vi "TwoBallShortAuton.vi"(11 "Intake Suck at Beginning?":bool) -> ()   [LabVIEW 2013]
uses:
  <vilib>/Rock Robotics/WPI/SafetyOutput/WPI_SafetyOutputConfigMenu.ctl
  <vilib>/Rock Robotics/WPI/Solenoid/WPI_SolenoidValue.ctl
  <vilib>/Rock Robotics/WPI/RobotDrive/WPI_RobotDriveGetSetRefNum.vi
  <vilib>/Rock Robotics/WPI/Solenoid/WPI_SolenoidSetEnum.vi
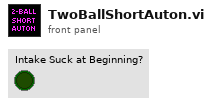
[diagram p1: front panel]
types:
  T1 = typedef "WPI_SafetyOutputConfigMenu.ctl" = enum16{"Enable", "Disable"}
  T2 = typedef "WPI_RobotDriveDevRef.ctl" = cluster{"DevStatus":errorcluster, "Motors[]":T3[], "Square Inputs":bool, "Max Output":dbl, "Isochronous":bool}
  T3 = typedef "WPI_MotorControlDeviceRef.ctl" = cluster{"DeviceStatus":errorcluster, "Type":enum16{"PWM", "CAN"}, "PWM":cluster{"Digital Module":T4, "PWM Channel":T5, "DeadBand":T6}, "CAN":cluster{"Device Number":u8, "Control Mode":T7, "Semaphore":T8, "Max Vout":dbl}, "Invert":bool, "TransformRef":T9, "InvTransformRef":T9}
  T4 = typedef "FPGA_TypedefDigitalModule.ctl" = enum16{"Digital Module 1", "Digital Module 2"}
  T5 = typedef "FPGA_DIOPWMChannel.ctl" = enum8{"PWM 1", "PWM 2", "PWM 3", "PWM 4", "PWM 5", "PWM 6", "PWM 7", "PWM 8", "PWM 9", "PWM 10", "Invalid"}
  T6 = typedef "WPI_PWMDeadband.ctl" = cluster{"Name":string, "maxPositivePwm":i32, "minPositivePwm":i32, "centerPwm":i32, "maxNegativePwm":i32, "minNegativePwm":i32, "angularRange":u16}
  T7 = typedef "WPI_CANJaguar_ControlMode.ctl" = enum8{"Percent VBus", "Current", "Speed", "Position", "Voltage"}
  T8 = typedef "Semaphore RefNum" = refnum<k1>
  T9 = typedef "WPI_PWMTransform_ConPane.ctl" = refnum<vi>
  T10 = typedef "WPI_DigitalInputDevRef.ctl" = cluster{"DevStatus":errorcluster, "DIO Channel":T11, "Digital Module":T4}
  T11 = typedef "FPGA_DIOChannel.ctl" = enum8{"DIO 1", "DIO 2", "DIO 3", "DIO 4", "DIO 5", "DIO 6", "DIO 7", "DIO 8", "DIO 9", "DIO 10", "DIO 11", "DIO 12", "DIO 13", "DIO 14", "Invalid"}
  T12 = typedef "WPI_SolenoidDevRef.ctl" = cluster{"DevStatus":errorcluster, "Solenoid Module":T13, "Forward Solenoid Channel":T14, "Reverse Solenoid Channel":T14}
  T13 = typedef "FPGA_TypedefSolenoidModule.ctl" = enum16{"Solenoid Module 1", "Solenoid Module 2"}
  T14 = typedef "WPI_SolenoidChannel.ctl" = enum8{"Solenoid 1", "Solenoid 2", "Solenoid 3", "Solenoid 4", "Solenoid 5", "Solenoid 6", "Solenoid 7", "Solenoid 8", "Invalid"}
  T15 = typedef "WPI_EncoderDevRef.ctl" = cluster{"DevStatus":errorcluster, "EncoderIndex":T16, "CounterIndex":T17, "DistancePerCount":dbl, "Decoding Type":T18}
  T16 = typedef "FPGA_EncoderIdx.ctl" = enum8{"Enc 0", "Enc 1", "Enc 2", "Enc 3", "Invalid"}
  T17 = typedef "FPGA_CounterCtrSystemIndex.ctl" = enum8{"Ctr 0", "Ctr 1", "Ctr 2", "Ctr 3", "Ctr 4", "Ctr 5", "Ctr 6", "Ctr 7", "Invalid"}
  T18 = typedef "WPI_EncoderType.ctl" = enum16{"1x", "2x", "4x"}
  T19 = typedef "WPI_SolenoidValue.ctl" = enum16{"Off", "On", "Forward", "Reverse"}
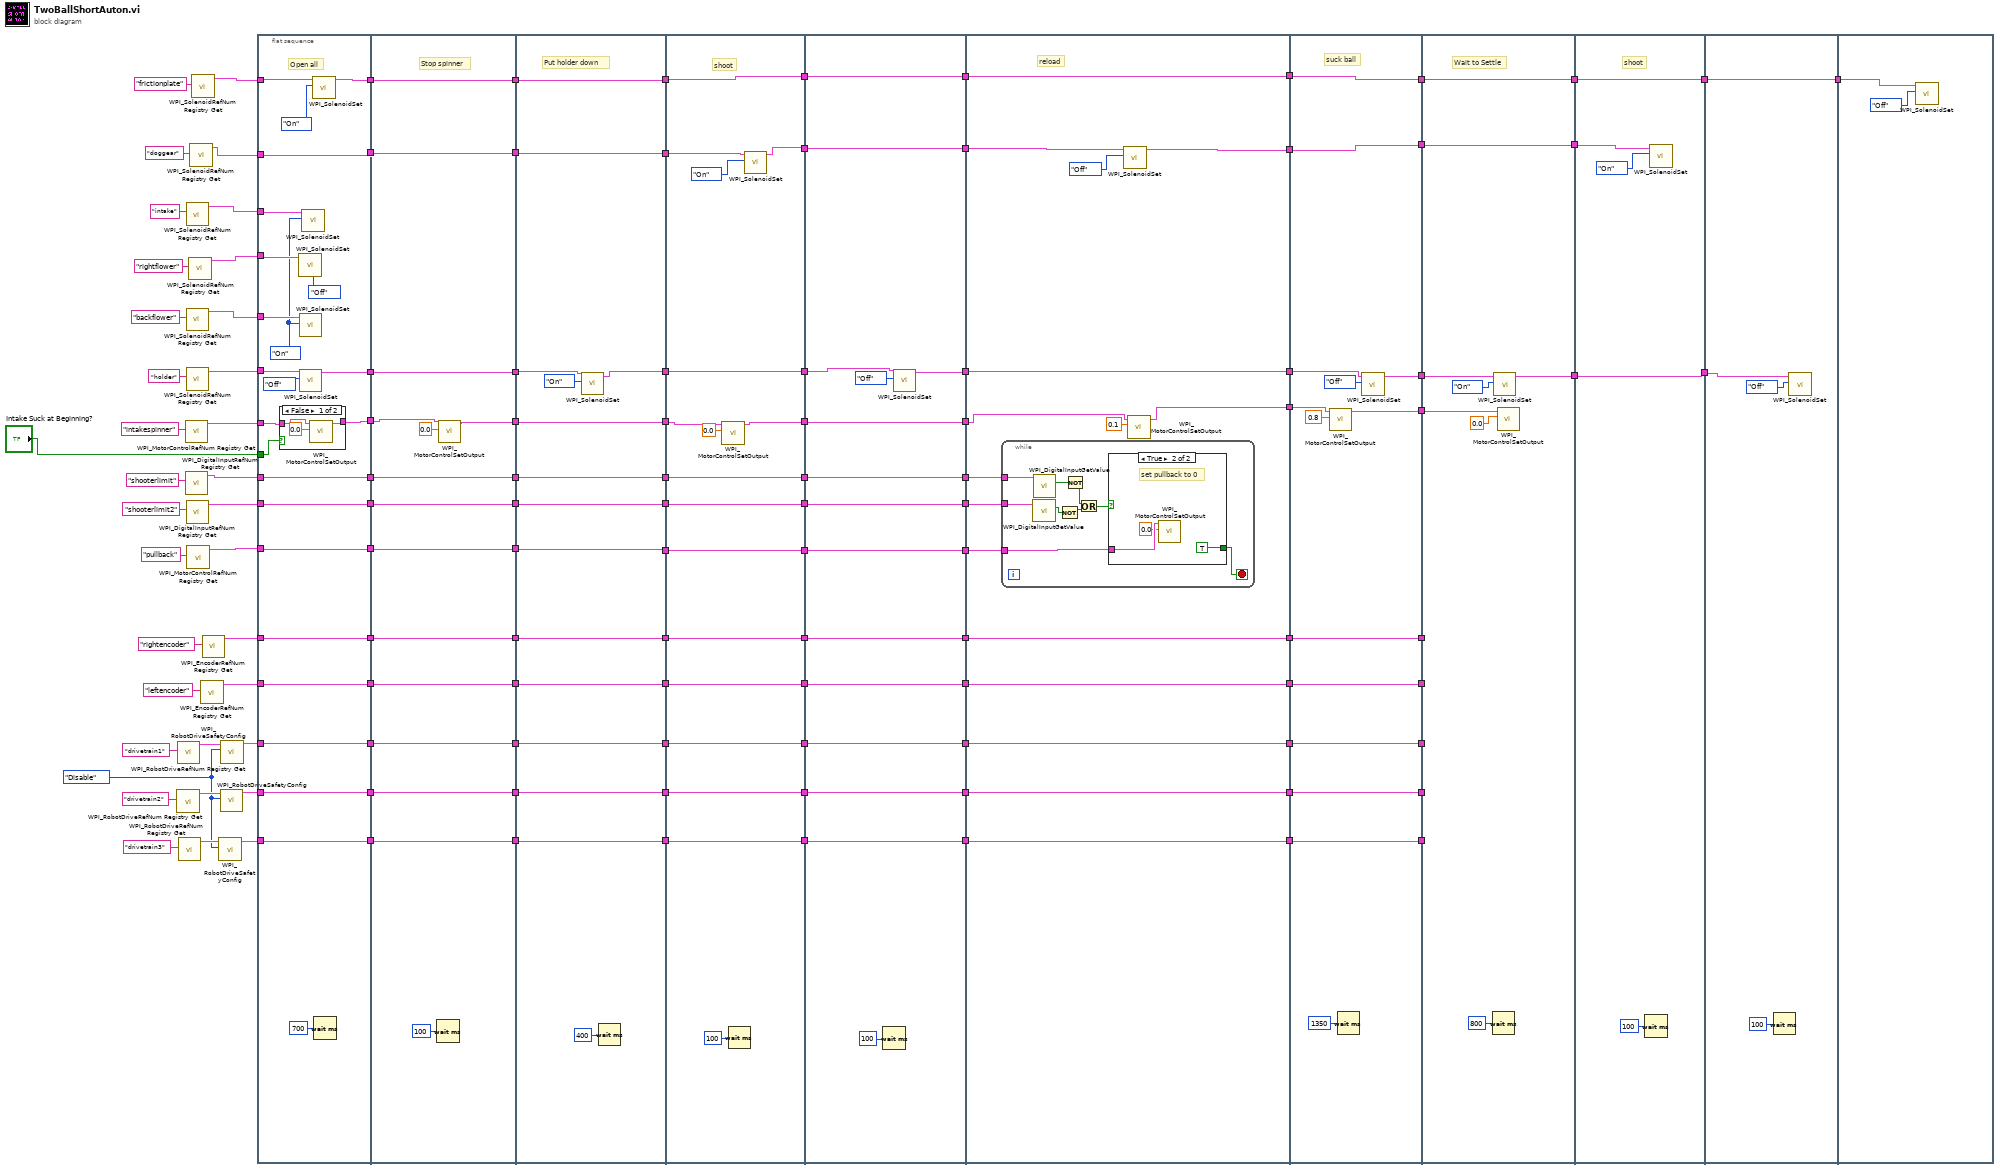
[diagram p0: block diagram]
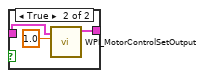
[diagram p2: hidden frame]
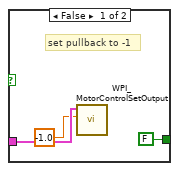
[diagram p3: hidden frame]
diagram:
  w41 = WPI_SafetyOutputConfigMenu."Disable" ("mode")
  n1 = call <vilib>:"WPI_RobotDriveRefNum Registry Get.vi"("refnum name"="drivetrain2") -> ("RobotDriveDevRef"=w43:T2)  [unwired: 9 in, 1 out]
  n2 = call <vilib>:"WPI_RobotDriveRefNum Registry Get.vi"("refnum name"="drivetrain1") -> ("RobotDriveDevRef"=w44:T2)  [unwired: 9 in, 1 out]
  n3 = call <vilib>:"WPI_RobotDriveRefNum Registry Get.vi"("refnum name"="drivetrain3") -> ("RobotDriveDevRef"=w42:T2)  [unwired: 9 in, 1 out]
  n4 = call <vilib>:"WPI_MotorControlRefNum Registry Get.vi"("refnum name"="intakespinner") -> ("MotorControlDevRef"=w54:T3)  [unwired: 9 in, 1 out]
  n5 = call <vilib>:"WPI_DigitalInputRefNum Registry Get.vi"("refnum name"="shooterlimit") -> ("DigitalInputDevRef"=w52:T10)  [unwired: 9 in, 1 out]
  n6 = call <vilib>:"WPI_SolenoidRefNum Registry Get.vi"("refnum name"="intake") -> ("SolenoidDevRef"=w58:T12)  [unwired: 9 in, 1 out]
  n7 = call <vilib>:"WPI_SolenoidRefNum Registry Get.vi"("refnum name"="backflower") -> ("SolenoidDevRef"=w56:T12)  [unwired: 9 in, 1 out]
  n8 = call <vilib>:"WPI_SolenoidRefNum Registry Get.vi"("refnum name"="holder") -> ("SolenoidDevRef"=w29:T12)  [unwired: 9 in, 1 out]
  n9 = call <vilib>:"WPI_DigitalInputRefNum Registry Get.vi"("refnum name"="shooterlimit2") -> ("DigitalInputDevRef"=w31:T10)  [unwired: 9 in, 1 out]
  n10 = call <vilib>:"WPI_MotorControlRefNum Registry Get.vi"("refnum name"="pullback") -> ("MotorControlDevRef"=w50:T3)  [unwired: 9 in, 1 out]
  n11 = call <vilib>:"WPI_SolenoidRefNum Registry Get.vi"("refnum name"="rightflower") -> ("SolenoidDevRef"=w57:T12)  [unwired: 9 in, 1 out]
  n12 = call <vilib>:"WPI_SolenoidRefNum Registry Get.vi"("refnum name"="doggear") -> ("SolenoidDevRef"=w62:T12)  [unwired: 9 in, 1 out]
  n13 = call <vilib>:"WPI_SolenoidRefNum Registry Get.vi"("refnum name"="frictionplate") -> ("SolenoidDevRef"=w33:T12)  [unwired: 9 in, 1 out]
  n14 = call <vilib>:"WPI_EncoderRefNum Registry Get.vi"("refnum name"="leftencoder") -> ("EncoderDevRef"=w39:T15)  [unwired: 9 in, 1 out]
  n15 = call <vilib>:"WPI_EncoderRefNum Registry Get.vi"("refnum name"="rightencoder") -> ("EncoderDevRef"=w40:T15)  [unwired: 9 in, 1 out]
  n16 = call <vilib>:"WPI_RobotDriveSafetyConfig.vi"("mode"=w41, "RobotDriveDevRef"=w42) -> ("RobotDriveDevRef"=w36:T2)  [unwired: 8 in, 1 out]
  n17 = call <vilib>:"WPI_RobotDriveSafetyConfig.vi"("mode"=w41, "RobotDriveDevRef"=w43) -> ("RobotDriveDevRef"=w37:T2)  [unwired: 8 in, 1 out]
  n18 = call <vilib>:"WPI_RobotDriveSafetyConfig.vi"("mode"=w41, "RobotDriveDevRef"=w44) -> ("RobotDriveDevRef"=w38:T2)  [unwired: 8 in, 1 out]
  n19 = flat-sequence {
    tunnel: w62 -> [w143]
    tunnel: [w143] -> w119
    tunnel: w58 -> [w142]
    tunnel: w57 -> [w141]
    tunnel: w56 -> [w140]
    tunnel: w54 -> [w138]
    tunnel: [w137] -> w118
    tunnel: w52 -> [w136]
    tunnel: [w136] -> w117
    tunnel: w50 -> [w135]
    tunnel: [w135] -> w116
    tunnel: [w134] -> w115
    tunnel: w40 -> [w134]
    tunnel: [w133] -> w114
    tunnel: w39 -> [w133]
    tunnel: [w132] -> w113
    tunnel: w38 -> [w132]
    tunnel: [w131] -> w112
    tunnel: w37 -> [w131]
    tunnel: [w130] -> w111
    tunnel: w36 -> [w130]
    tunnel: "Intake Suck at Beginning?" -> [w127]
    tunnel: w33 -> [w125]
    tunnel: [w124] -> w110
    tunnel: w31 -> [w123]
    tunnel: [w123] -> w109
    tunnel: w29 -> [w122]
    tunnel: [w120] -> w108
    tunnel: w119 -> [w164]
    tunnel: [w164] -> w107
    tunnel: w118 -> [w152]
    tunnel: w117 -> [w163]
    tunnel: [w163] -> w106
    tunnel: w116 -> [w162]
    tunnel: [w162] -> w105
    tunnel: w115 -> [w161]
    tunnel: [w161] -> w104
    tunnel: w114 -> [w160]
    tunnel: [w160] -> w103
    tunnel: w113 -> [w159]
    tunnel: [w159] -> w102
    tunnel: w112 -> [w158]
    tunnel: [w158] -> w101
    tunnel: w111 -> [w157]
    tunnel: [w157] -> w100
    tunnel: w110 -> [w156]
    tunnel: [w156] -> w99
    tunnel: w109 -> [w155]
    tunnel: [w155] -> w98
    tunnel: w108 -> [w154]
    tunnel: [w154] -> w97
    tunnel: [w151] -> w96
    tunnel: [w166] -> w95
    tunnel: [w178] -> w94
    tunnel: [w177] -> w93
    tunnel: [w176] -> w92
    tunnel: [w175] -> w91
    tunnel: [w174] -> w90
    tunnel: [w173] -> w89
    tunnel: [w172] -> w88
    tunnel: [w171] -> w87
    tunnel: [w170] -> w86
    tunnel: [w169] -> w85
    tunnel: [w167] -> w84
    tunnel: w107 -> [w176]
    tunnel: w106 -> [w178]
    tunnel: w105 -> [w177]
    tunnel: w104 -> [w174]
    tunnel: w103 -> [w175]
    tunnel: w102 -> [w173]
    tunnel: w101 -> [w172]
    tunnel: w100 -> [w171]
    tunnel: w99 -> [w170]
    tunnel: w98 -> [w169]
    tunnel: w97 -> [w165]
    tunnel: w96 -> [w166]
    tunnel: w95 -> [w194]
    tunnel: [w193] -> w28
    tunnel: w94 -> [w196]
    tunnel: [w196] -> w26
    tunnel: w93 -> [w195]
    tunnel: [w195] -> w24
    tunnel: [w189] -> w22
    tunnel: w92 -> [w188]
    tunnel: [w187] -> w20
    tunnel: w91 -> [w187]
    tunnel: [w186] -> w18
    tunnel: w90 -> [w186]
    tunnel: [w185] -> w16
    tunnel: w89 -> [w185]
    tunnel: [w184] -> w14
    tunnel: w88 -> [w184]
    tunnel: [w183] -> w12
    tunnel: w87 -> [w183]
    tunnel: w86 -> [w182]
    tunnel: [w182] -> w10
    tunnel: w85 -> [w181]
    tunnel: [w181] -> w8
    tunnel: w84 -> [w180]
    tunnel: [w180] -> w6
    tunnel: w28 -> [w211]
    tunnel: [w211] -> w27
    tunnel: w26 -> [w210]
    tunnel: [w210] -> w25
    tunnel: w24 -> [w209]
    tunnel: [w209] -> w23
    tunnel: w22 -> [w208]
    tunnel: [w208] -> w21
    tunnel: w20 -> [w207]
    tunnel: [w207] -> w19
    tunnel: w18 -> [w206]
    tunnel: [w206] -> w17
    tunnel: w16 -> [w205]
    tunnel: [w205] -> w15
    tunnel: w14 -> [w204]
    tunnel: [w204] -> w13
    tunnel: w12 -> [w203]
    tunnel: [w203] -> w11
    tunnel: w10 -> [w202]
    tunnel: [w202] -> w9
    tunnel: w8 -> [w201]
    tunnel: [w201] -> w7
    tunnel: w6 -> [w199]
    tunnel: [w198] -> w5
    tunnel: w27 -> [w213]
    tunnel: w25 -> [w227]
    tunnel: w23 -> [w226]
    tunnel: [w224] -> w83
    tunnel: w21 -> [w223]
    tunnel: [w222] -> w82
    tunnel: w19 -> [w222]
    tunnel: [w221] -> w81
    tunnel: w17 -> [w221]
    tunnel: [w220] -> w80
    tunnel: w15 -> [w220]
    tunnel: [w219] -> w79
    tunnel: w13 -> [w219]
    tunnel: [w218] -> w78
    tunnel: w11 -> [w218]
    tunnel: w9 -> [w217]
    tunnel: [w217] -> w77
    tunnel: w7 -> [w216]
    tunnel: w5 -> [w215]
    tunnel: [w215] -> w76
    tunnel: [w212] -> w75
    tunnel: [w256] -> w68
    tunnel: [w253] -> w69
    tunnel: w83 -> [w256]
    tunnel: w82 -> [w251]
    tunnel: w81 -> [w252]
    tunnel: [w252] -> w70
    tunnel: [w251] -> w71
    tunnel: [w250] -> w72
    tunnel: w80 -> [w250]
    tunnel: [w249] -> w73
    tunnel: w79 -> [w249]
    tunnel: [w248] -> w74
    tunnel: w78 -> [w248]
    tunnel: [w247] -> w67
    tunnel: w77 -> [w247]
    tunnel: w76 -> [w245]
    tunnel: [w244] -> w66
    tunnel: w75 -> [w243]
    tunnel: [w264] -> w64
    tunnel: w74 -> [_]
    tunnel: w73 -> [_]
    tunnel: w72 -> [_]
    tunnel: w71 -> [_]
    tunnel: w70 -> [_]
    tunnel: w69 -> [w261]
    tunnel: w68 -> [w264]
    tunnel: w67 -> [w260]
    tunnel: [w260] -> w65
    tunnel: w66 -> [w259]
    tunnel: [w257] -> w1
    tunnel: [w266] -> w4
    tunnel: w65 -> [w266]
    tunnel: w64 -> [w267]
    tunnel: [w265] -> w2
    tunnel: w1 -> [w265]
    tunnel: w4 -> [w273]
    tunnel: [w273] -> w3
    tunnel: w2 -> [w271]
    tunnel: w3 -> [w274]
    frame #0 {
      w129 = WPI_SolenoidValue."On" ("Value")
      # "Open all"
      n20 = case shown="False" w127 {
        tunnel: w138 -> [w145 w149]
        tunnel: [w144 w147] -> w137
        frame False {
          n21 = call <vilib>:"WPI_MotorControlSetOutput.vi"("Output"=0.0, "MotorControlDevRef"=w145) -> ("MotorControlDevRef"=w144:T3)  [unwired: 7 in, 2 out]
        }
        frame True {
          n22 = call <vilib>:"WPI_MotorControlSetOutput.vi"("Output"=1.0, "MotorControlDevRef"=w149) -> ("MotorControlDevRef"=w147:T3)  [unwired: 7 in, 2 out]
        }
      }
      n23 = call-poly <vilib>:"WPI_SolenoidSet.vi"("Value"=WPI_SolenoidValue."Off", "SolenoidDevRef"=w141) -> ()  [unwired: 8 in, 2 out]
      n24 = call-poly <vilib>:"WPI_SolenoidSet.vi"("Value"=w129, "SolenoidDevRef"=w140) -> ()  [unwired: 8 in, 2 out]
      n25 = call-poly <vilib>:"WPI_SolenoidSet.vi"("Value"=WPI_SolenoidValue."Off", "SolenoidDevRef"=w122) -> ("SolenoidDevRef"=w120:T12)  [unwired: 8 in, 1 out]
      n26 = call-poly <vilib>:"WPI_SolenoidSet.vi"("Value"=w129, "SolenoidDevRef"=w142) -> ()  [unwired: 8 in, 2 out]
      n27 = call-poly <vilib>:"WPI_SolenoidSet.vi"("Value"=WPI_SolenoidValue."On", "SolenoidDevRef"=w125) -> ("SolenoidDevRef"=w124:T12)  [unwired: 8 in, 1 out]
      n28 = Wait (ms)(milliseconds to wait=u32 700) -> ()  [unwired: 1 out]
    }
    frame #1 {
      # "Stop spinner"
      n29 = Wait (ms)(milliseconds to wait=u32 100) -> ()  [unwired: 1 out]
      n30 = call <vilib>:"WPI_MotorControlSetOutput.vi"("Output"=0.0, "MotorControlDevRef"=w152) -> ("MotorControlDevRef"=w151:T3)  [unwired: 7 in, 2 out]
    }
    frame #2 {
      # "Put holder down"
      n31 = call-poly <vilib>:"WPI_SolenoidSet.vi"("Value"=WPI_SolenoidValue."On", "SolenoidDevRef"=w165) -> ("SolenoidDevRef"=w167:T12)  [unwired: 8 in, 1 out]
      n32 = Wait (ms)(milliseconds to wait=u32 400) -> ()  [unwired: 1 out]
    }
    frame #3 {
      # "shoot"
      n33 = call <vilib>:"WPI_MotorControlSetOutput.vi"("Output"=0.0, "MotorControlDevRef"=w194) -> ("MotorControlDevRef"=w193:T3)  [unwired: 7 in, 2 out]
      n34 = Wait (ms)(milliseconds to wait=u32 100) -> ()  [unwired: 1 out]
      n35 = call-poly <vilib>:"WPI_SolenoidSet.vi"("Value"=WPI_SolenoidValue."On", "SolenoidDevRef"=w188) -> ("SolenoidDevRef"=w189:T12)  [unwired: 8 in, 1 out]
    }
    frame #4 {
      n36 = Wait (ms)(milliseconds to wait=u32 100) -> ()  [unwired: 1 out]
      n37 = call-poly <vilib>:"WPI_SolenoidSet.vi"("Value"=WPI_SolenoidValue."Off", "SolenoidDevRef"=w199) -> ("SolenoidDevRef"=w198:T12)  [unwired: 8 in, 1 out]
    }
    frame #5 {
      # "reload"
      n38 = while {
        tunnel: w227 -> [w236]
        tunnel: w226 -> [w234]
        tunnel: w216 -> [w232]
        stop <- w233 stop-if-true
        n39 = call <vilib>:"WPI_DigitalInputGetValue.vi"("DigitalInputDevRef"=w232) -> ("Value"=w228:bool)  [unwired: 8 in, 2 out]
        n40 = call <vilib>:"WPI_DigitalInputGetValue.vi"("DigitalInputDevRef"=w236) -> ("Value"=w235:bool)  [unwired: 8 in, 2 out]
        n41 = Not(x=w228) -> (.not. x?=w229:bool)
        n42 = Not(x=w235) -> (.not. x?=w231:bool)
        n43 = Or(x=w231, y=w229) -> (x .or. y?=w230:bool)
        n44 = case shown="True" w230 {
          tunnel: w234 -> [w239 w242]
          tunnel: [FALSE TRUE] -> w233
          frame False {
            # "set pullback to -1"
            n45 = call <vilib>:"WPI_MotorControlSetOutput.vi"("Output"=-1.0, "MotorControlDevRef"=w239) -> ()  [unwired: 7 in, 3 out]
          }
          frame True {
            # "set pullback to 0"
            n46 = call <vilib>:"WPI_MotorControlSetOutput.vi"("Output"=0.0, "MotorControlDevRef"=w242) -> ()  [unwired: 7 in, 3 out]
          }
        }
      }
      n47 = call-poly <vilib>:"WPI_SolenoidSet.vi"("Value"=WPI_SolenoidValue."Off", "SolenoidDevRef"=w223) -> ("SolenoidDevRef"=w224:T12)  [unwired: 8 in, 1 out]
      n48 = call <vilib>:"WPI_MotorControlSetOutput.vi"("Output"=0.1, "MotorControlDevRef"=w213) -> ("MotorControlDevRef"=w212:T3)  [unwired: 7 in, 2 out]
    }
    frame #6 {
      # "suck ball"
      n49 = call <vilib>:"WPI_MotorControlSetOutput.vi"("Output"=0.8, "MotorControlDevRef"=w243) -> ("MotorControlDevRef"=w253:T3)  [unwired: 7 in, 2 out]
      n50 = Wait (ms)(milliseconds to wait=u32 1350) -> ()  [unwired: 1 out]
      n51 = call-poly <vilib>:"WPI_SolenoidSet.vi"("Value"=WPI_SolenoidValue."Off", "SolenoidDevRef"=w245) -> ("SolenoidDevRef"=w244:T12)  [unwired: 8 in, 1 out]
    }
    frame #7 {
      # "Wait to Settle"
      n52 = Wait (ms)(milliseconds to wait=u32 800) -> ()  [unwired: 1 out]
      n53 = call-poly <vilib>:"WPI_SolenoidSet.vi"("Value"=WPI_SolenoidValue."On", "SolenoidDevRef"=w259) -> ("SolenoidDevRef"=w257:T12)  [unwired: 8 in, 1 out]
      n54 = call <vilib>:"WPI_MotorControlSetOutput.vi"("Output"=0.0, "MotorControlDevRef"=w261) -> ()  [unwired: 7 in, 3 out]
    }
    frame #8 {
      # "shoot"
      n55 = Wait (ms)(milliseconds to wait=u32 100) -> ()  [unwired: 1 out]
      n56 = call-poly <vilib>:"WPI_SolenoidSet.vi"("Value"=WPI_SolenoidValue."On", "SolenoidDevRef"=w267) -> ()  [unwired: 8 in, 2 out]
    }
    frame #9 {
      n57 = Wait (ms)(milliseconds to wait=u32 100) -> ()  [unwired: 1 out]
      n58 = call-poly <vilib>:"WPI_SolenoidSet.vi"("Value"=WPI_SolenoidValue."Off", "SolenoidDevRef"=w271) -> ()  [unwired: 8 in, 2 out]
    }
    frame #10 {
      n59 = call-poly <vilib>:"WPI_SolenoidSet.vi"("Value"=WPI_SolenoidValue."Off", "SolenoidDevRef"=w274) -> ()  [unwired: 8 in, 2 out]
    }
  }
